vi "spikePositionGraph.vi"() -> ()   [LabVIEW 2025, in "spikeController.lvclass"]
uses:
  spikeController.lvclass
  spikeController.lvclass/spikeController.ctl
panel:
  out "Spike Position \n(via Potentiometer)":dbl[](graph)
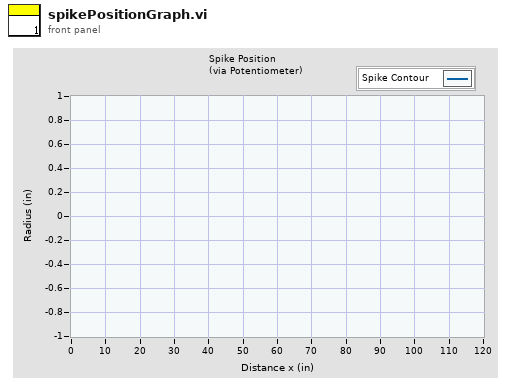
[diagram p1: front panel]
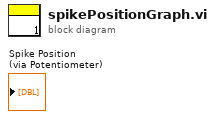
[diagram p0: block diagram]
diagram:
